vi "FGV Zustaende Loggen.vi"(6 "Aktionen Zustände Loggen":T2, 7 "Sprachliste":string[][](array[string]), 8 "Herkunft":string="---", 10 "Zustand ALT":T1, 11 "Zustand NEU":T1) -> (2 "Log Daten Lang":string[](array[string]), 3 "Log Daten":string[](array[string]))   [LabVIEW 2020, in "Funktionstasten.lvlib"]
uses:
  Funktionstasten.lvlib
  Aktionen Zustaende Loggen.ctl
  Zustaende.ctl
  SysLog/SysLog Interface.ctl
  Allgemein/allgemeine Sub-VIs.lvlib
  SysLog/SysLog.lvlib
  Sprachverwaltung/Sprachverwaltung.lvlib
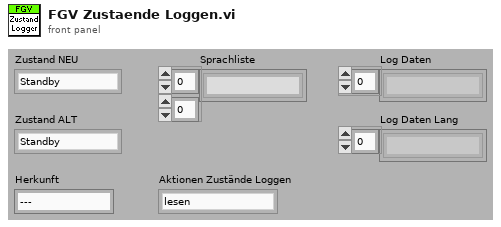
[diagram p1: front panel]
types:
  T1 = typedef "Funktionstasten.lvlib/Zustaende.ctl" = enum16{"Standby", "Pause", "Eco", "Messen", "Kalibrieren", "Spülen Filter", "Spülen Leitung", "Umgebungsluft", "0-Gas", "Cal-Gas", "CG zu PNS", "-------------", "Init 1", "Init 2", "Init 3", "Init 4", "Messen vorbereiten", "Messen durchführen", "Exit"}
  T2 = typedef "Funktionstasten.lvlib/Aktionen Zustaende Loggen.ctl" = enum16{"lesen", "schreiben", "löschen", "init"}
  T3 = typedef "SysLog.lvlib/SysLog Interface.ctl" = cluster{"FehlermeldungsCode":i32, "ErfolgsmeldungsCode":i32, "ParameterListenString":string, "Anzeige":bool, "SysLogIcon":enum16{"OK", "Warnung", "Fehler"}, "intern":bool}
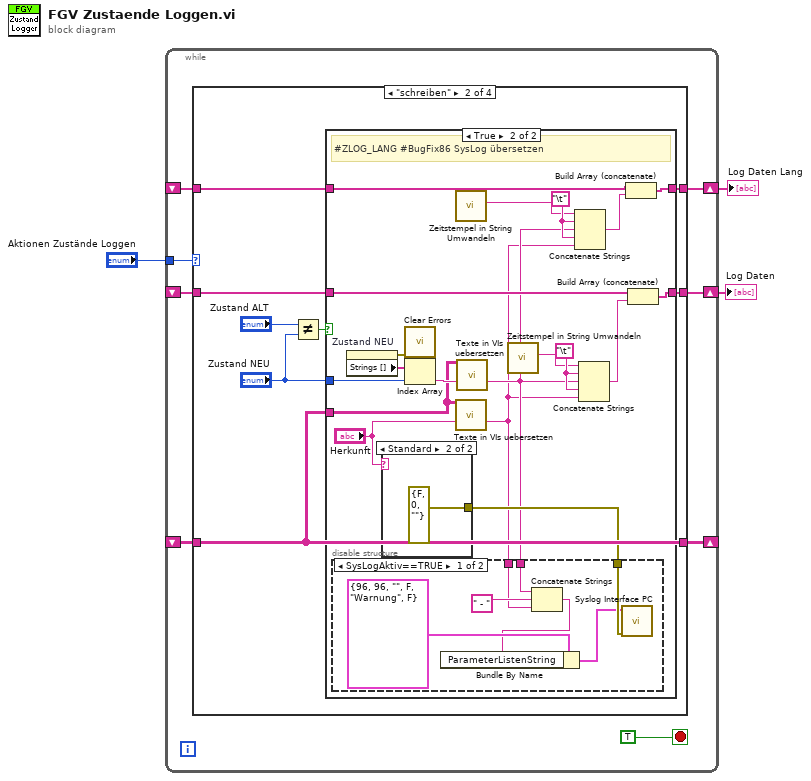
[diagram p0: block diagram]
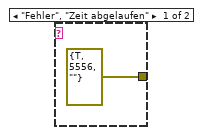
[diagram p5: hidden frame]
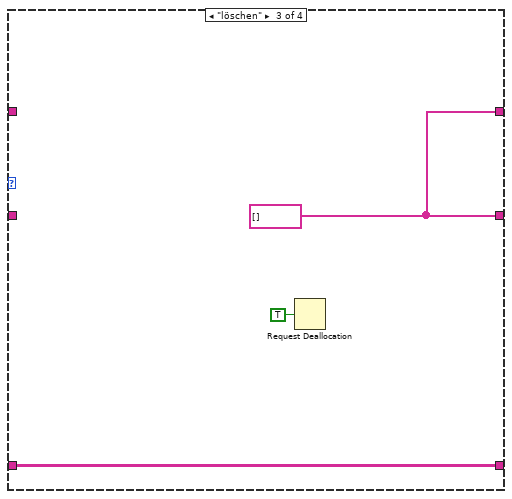
[diagram p6: hidden frame]
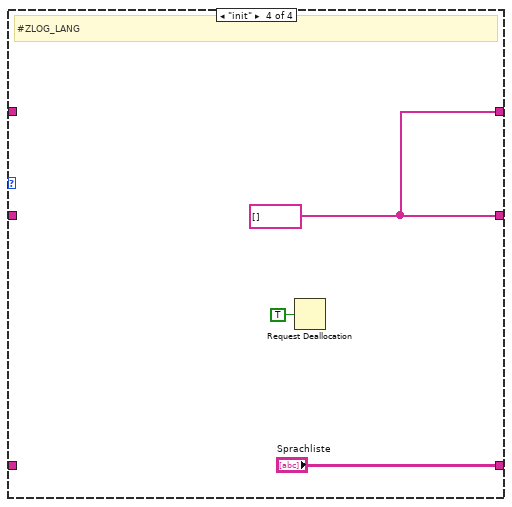
[diagram p7: hidden frame]
diagram:
  n1 = while {
    tunnel: "Aktionen Zustände Loggen" -> [w10]
    shift-right: [w9] -> w2
    shift-left: _ -> [w8]
    shift-right: [w7] -> _
    shift-left: _ -> [w6]
    shift-right: [w5] -> w1
    shift-left: _ -> [w4]
    stop <- TRUE stop-if-true
    n2 = case shown="\"schreiben\"" w10 {
      tunnel: [w14 w22 w53 w56] -> w9
      tunnel: w8 -> [w14 w21 _ _]
      tunnel: [w13 w17 w54 "Sprachliste"] -> w7
      tunnel: w6 -> [w13 w17 w54 _]
      tunnel: [w12 w16 w53 w56] -> w5
      tunnel: w4 -> [w12 w15 _ _]
      frame "lesen", Default {
      }
      frame "schreiben" {
        n3 = Not Equal?(x="Zustand ALT", y="Zustand NEU") -> (x != y?=w20:bool)
        n4 = case shown="True" w20 {
          tunnel: "Zustand NEU" -> [_ w42]
          tunnel: [w24 w38] -> w22
          tunnel: w21 -> [w24 w36]
          tunnel: w17 -> [_ w27]
          tunnel: [w23 w29] -> w16
          tunnel: w15 -> [w23 w28]
          frame False {
          }
          frame True {
            w32 = "\t"
            w41 = "\t"
            # "#ZLOG_LANG #BugFix86 SysLog übersetzen"
            n5 = property on="Zustand NEU" class="Enum (strikt)"() -> (error out=w37:errorcluster, "Strings []"=w43:string[])  [unwired: 2 in, 1 out]
            n6 = case shown="Standard" "Herkunft" {
              tunnel: [errorcluster {"status"=TRUE, "code"=5556, "source"=""} ("Fehler (in)") errorcluster {"status"=FALSE, "code"=0, "source"=""} ("Fehler (in)")] -> w35
              frame "Fehler", "Zeit abgelaufen" {
              }
              frame Default {
              }
            }
            n7 = call <vilib>:"Clear Errors.vi"("error in (no error)"=w37) -> ()  [unwired: 5 in, 2 out]
            n8 = Index Array(array=w43, index=w42) -> (element=w34:string)
            n9 = call "Zeitstempel in String Umwandeln.vi"() -> ("Zeitstempel mit Kommastellen"=w31:string)  [unwired: 10 in, 1 out]
            n10 = call "Texte in VIs uebersetzen.vi"("Sprachliste"=w27, "String zum Übersetzen"="Herkunft") -> ("String zum Übersetzen"=w25:string)  [unwired: 9 in, 4 out]
            n11 = call "Texte in VIs uebersetzen.vi"("Sprachliste"=w27, "String zum Übersetzen"=w34) -> ("String zum Übersetzen"=w26:string)  [unwired: 9 in, 4 out]
            n12 = disable-structure shown="SysLogAktiv==TRUE" {
              disable-tunnel: w26 -> [w49 _]
              disable-tunnel: w25 -> [w48 _]
              disable-tunnel: w35 -> [w47 _]
              frame condition #0 (active) {
                n13 = Concatenate Strings(w49, " - ", w48) -> (w45:string)
                n14 = Bundle By Name(cluster=T3 {"FehlermeldungsCode"=96, "ErfolgsmeldungsCode"=96, "ParameterListenString"="", "Anzeige"=FALSE, "SysLogIcon"=enum."Warnung", "intern"=FALSE} ("Cluster (in)"), "ParameterListenString"=w45) -> (w44:T3)
                n15 = call "Syslog Interface PC.vi"("Fehler (in)"=w47, "Cluster (in)"=w44) -> ()  [unwired: 9 in, 1 out]
              }
              frame condition #1 {
              }
            }
            n16 = call "Zeitstempel in String Umwandeln.vi"() -> ("Zeitstempel mit Kommastellen"=w40:string)  [unwired: 10 in, 1 out]
            n17 = Concatenate Strings(w31, w32, w26, w32, w25) -> (w30:string)
            n18 = Concatenate Strings(w40, w41, w26, w41, w25) -> (w39:string)
            n19 = Build Array (concatenate)(w28, w30) -> (w29:string[])
            n20 = Build Array (concatenate)(w36, w39) -> (w38:string[])
          }
        }
      }
      frame "löschen" {
        w53 = string[] []
        n21 = Request Deallocation(TRUE ("Flag")) -> ()
      }
      frame "init" {
        w56 = string[] []
        # "#ZLOG_LANG"
        n22 = Request Deallocation(TRUE ("Flag")) -> ()
      }
    }
  }
  "Log Daten" <- w2
  "Log Daten Lang" <- w1
